vi "Processor LEH.vi"(7 "SimError":bool, 8 "error in":errorcluster) -> (0 "error out":errorcluster)   [LabVIEW 2018]
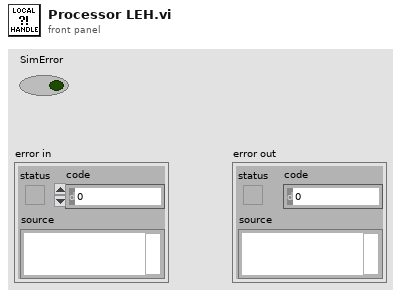
[diagram p1: front panel]
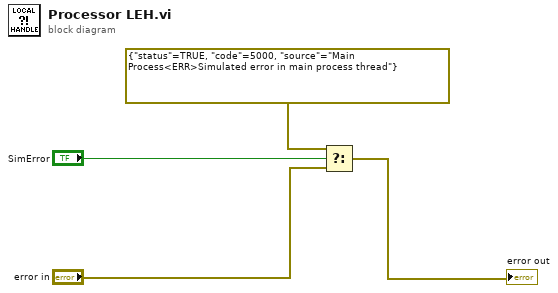
[diagram p0: block diagram]
diagram:
  n1 = Select(t=errorcluster {"status"=TRUE, "code"=5000, "source"="Main Process<ERR>Simulated error in main process thread"} ("error in"), s="SimError", f="error in") -> (s? t:f=→"error out":errorcluster)
